vi "workbook set custom property integer.vi"(8 "error in (no error)":errorcluster, 9 "value":i32, 10 "name":string, 11 "workbook":u32) -> (0 "error out":errorcluster, 3 "function return":u32(ring))   [LabVIEW 8.6]
doc: "lxw_error workbook_set_custom_property_integer(lxw_workbook workbook, const char *name, int32_t value);"
uses:
  pending_lvxlsxwriter/xlsxwriter.dll
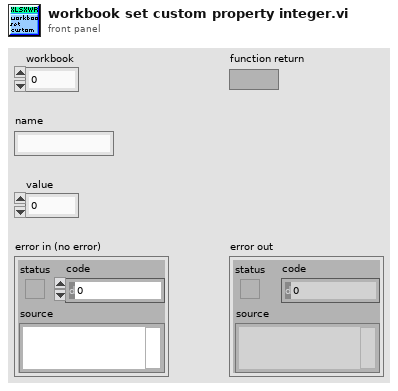
[diagram p1: front panel]
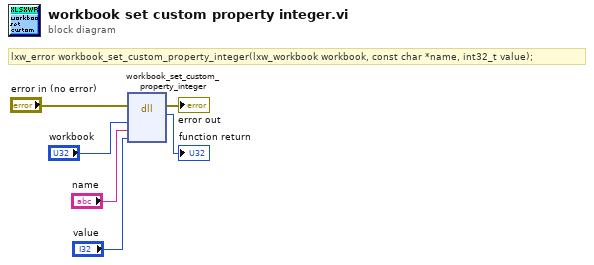
[diagram p0: block diagram]
diagram:
  # "lxw_error workbook_set_custom_property_integer(lxw_workbook workbook, const char *name, int32_t value);"
  n1 = dll-call lib="C:/Users/WDAGUtilityAccount/Desktop/pending_lvxlsxwriter/xlsxwriter.*" fn="workbook_set_custom_property_integer"(error in="error in (no error)", "workbook"="workbook", "name"="name", "value"="value") -> (error out=→"error out":errorcluster, →"function return":u32)  [unwired: 5 in, 1 out]
